vi "Encoders Per Iteration Calculator.vi"(3 "motor speed":dbl, 4 "total iterations":dbl, 5 "encoder count":dbl, 6 "go":bool) -> (0 "iterations":dbl, 1 "motor speed out":dbl, 2 "encoder counts per iteration":dbl)   [LabVIEW 2014]
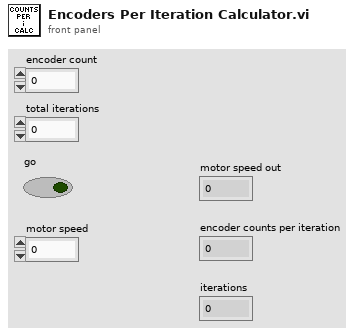
[diagram p1: front panel]
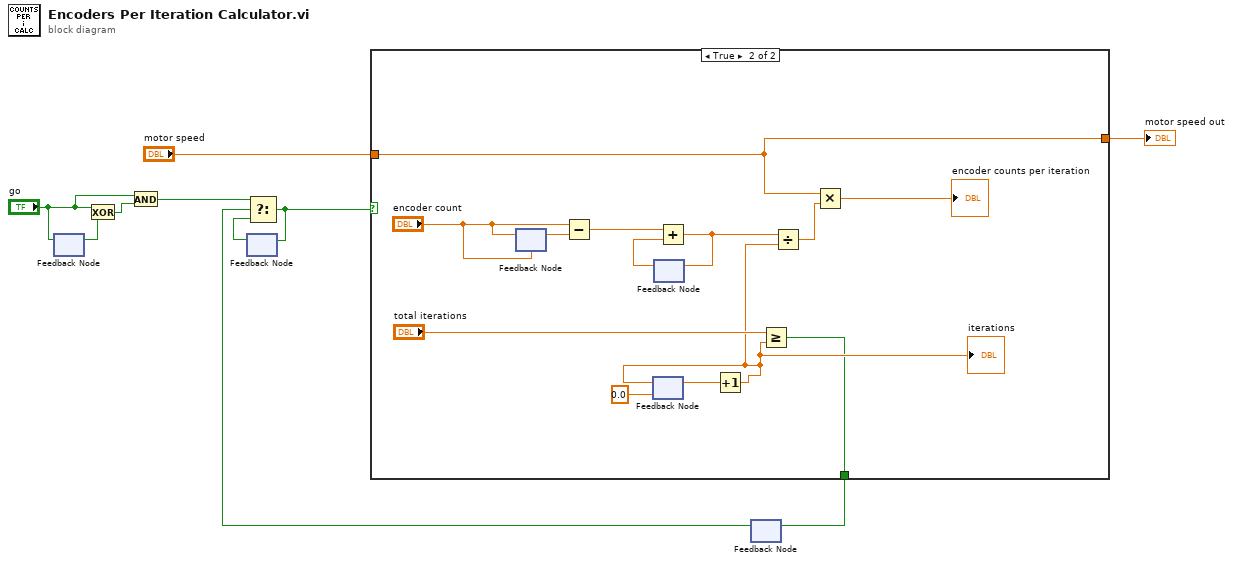
[diagram p0: block diagram]
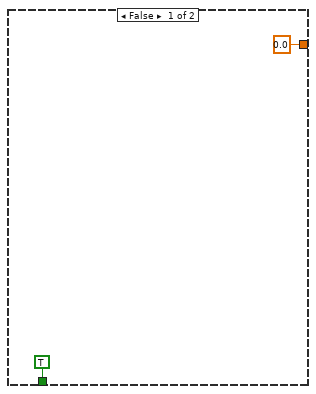
[diagram p2: hidden frame]
diagram:
  n1 = feedback-in #1("go") -> ()
  n2 = feedback #1() -> (w5:bool)  [unwired: 1 in]
  n3 = Exclusive Or(1:w5, 2:"go") -> (0:w4:bool)
  n4 = And(x="go", y=w4) -> (x .and. y?=w2:bool)
  n5 = feedback #2() -> (w7:bool)  [unwired: 1 in]
  n6 = feedback #3() -> (w8:bool)  [unwired: 1 in]
  n7 = Select(t=w2, s=w8, f=w7) -> (s? t:f=w6:bool)
  n8 = feedback-in #2(w6) -> ()
  n9 = case shown="True" w6 {
    tunnel: "motor speed" -> [_ w13]
    tunnel: [TRUE w14] -> w9
    tunnel: [0.0 ("motor speed") w13] -> w1
    frame False {
    }
    frame True {
      n10 = feedback #4("encoder count") -> (w22:dbl)
      n11 = feedback-in #4("encoder count") -> ()
      n12 = Subtract(x="encoder count", y=w22) -> (x-y=w21:dbl)
      n13 = feedback #5(0.0) -> (w24:dbl)
      n14 = feedback #6() -> (w20:dbl)  [unwired: 1 in]
      n15 = Add(x=w21, y=w20) -> (x+y=w19:dbl)
      n16 = feedback-in #6(w19) -> ()
      n17 = Increment(x=w24) -> (x+1=w18:dbl)
      "iterations" <- w18
      n18 = feedback-in #5(w18) -> ()
      n19 = Greater Or Equal?(x="total iterations", y=w18) -> (x >= y?=w14:bool)
      n20 = Divide(x=w19, y=w18) -> (x/y=w17:dbl)
      n21 = Multiply(x=w13, y=w17) -> (x*y=→"encoder counts per iteration":dbl)
    }
  }
  "motor speed out" <- w1
  n22 = feedback-in #3(w9) -> ()
